vi "EssaisRealises.vi"(3 "entrée d'erreur (pas d'erreur)":errorcluster caption="sortie d'erreur", 4 "WhichPath?":T1=enum."MeasTDMS", 5 "NomProjet":string) -> (0 "sortie d'erreur":errorcluster caption="error out", 2 "InfosFichiers":string[][](array[string]))   [LabVIEW 2017]
uses:
  DefDeType/WhichPath.ctl
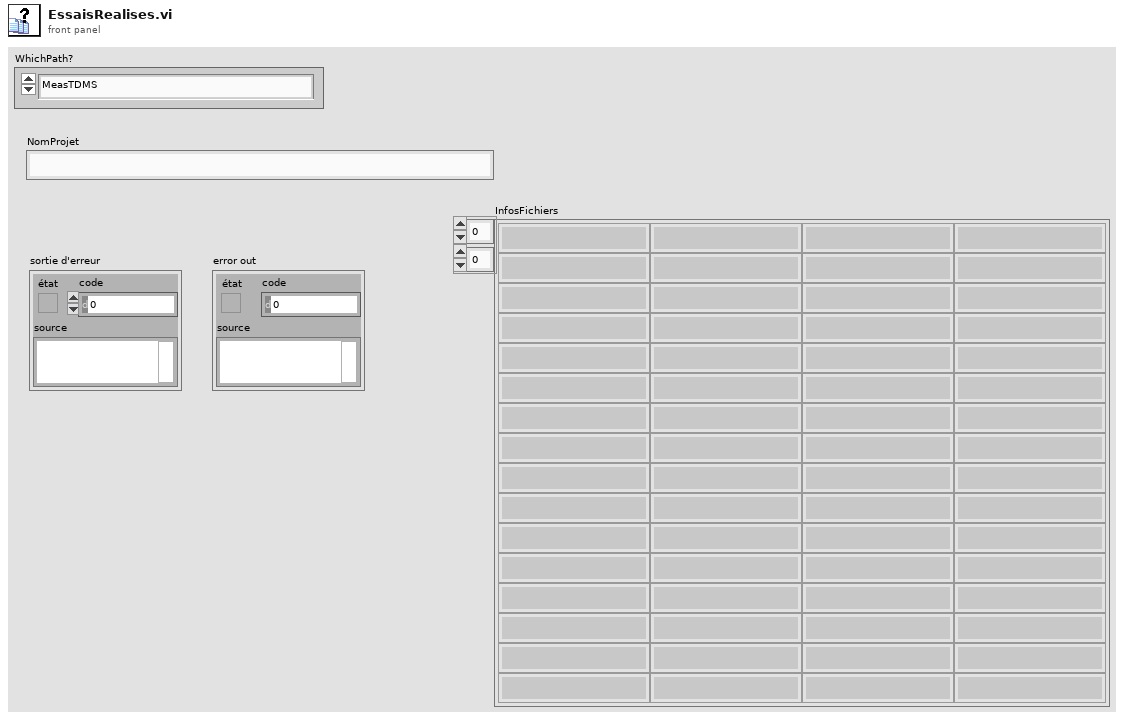
[diagram p1: front panel]
types:
  T1 = typedef "WhichPath.ctl" = enum16{"DossierProjet", "Config", "Meas", "MeasPCI", "MeasCRIO1", "MeasCRIO2", "MeasQualisys", "MeasHBM", "MeasTDMS", "Fig", "Res"}
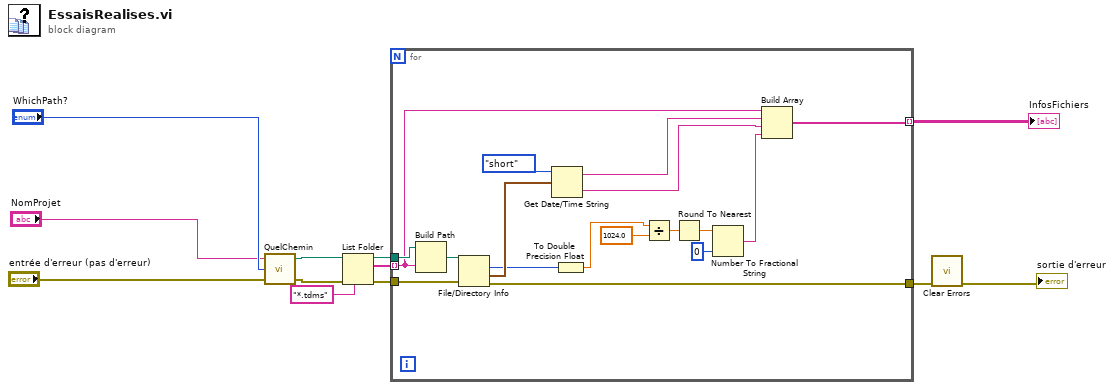
[diagram p0: block diagram]
diagram:
  n1 = call "QuelChemin.vi"("Entrée d'erreur"="entrée d'erreur (pas d'erreur)", "WhichPath?"="WhichPath?", "NomProjet"="NomProjet") -> ("Sortie d'erreur"=w6:errorcluster, "SurDisqueLocal"=w7:path)  [unwired: 1 out]
  n2 = List Folder(path=w7, pattern="*.tdms" ("filtre"), error in=w6) -> (path out=w11:path, filenames=w10:string[], error out=w9:errorcluster)  [unwired: 1 in, 1 out]
  n3 = for {
    tunnel: w9 -> [w28]
    tunnel: w10 -> [w18] mode=indexing
    tunnel: w11 -> [w29]
    tunnel: [w24] -> w12
    tunnel: [w14] -> w3 mode=indexing
    n4 = Build Path(base path=w29, name or relative path=w18) -> (appended path=w27:path)
    n5 = File/Directory Info(path=w27, error in=w28) -> (size=w22:i64, last mod=w26:timestamp, error out=w24:errorcluster)  [unwired: 4 out]
    n6 = Get Date/Time String(date format (0)=enum16{"short", "long", "abbreviated"}."short" ("format de date (0)"), seconds (now)=w26) -> (date string=w17:string, time string=w16:string)  [unwired: 1 in]
    n7 = To Double Precision Float(number=w22) -> (double precision float=w21:dbl)
    n8 = Divide(x=w21, y=1024.0) -> (x/y=w20:dbl)
    n9 = Round To Nearest(number=w20) -> (nearest integer value=w19:dbl)
    n10 = Number To Fractional String(number=w19, precision (6)=i16 0 ("précision (6)")) -> (F-format string=w15:string)  [unwired: 2 in]
    n11 = Build Array(w18, w17, w16, w15) -> (w14:string[])
  }
  "InfosFichiers" <- w3
  n12 = call <vilib>:"Clear Errors.vi"("error in (no error)"=w12) -> ("error out"=→"sortie d'erreur":errorcluster)  [unwired: 5 in, 1 out]
